vi "Initialize.vi"(7 "Serial Configuration":T1={"Baud Rate"=9600, "Parity"=0, "Data Bits"=8, "Stop Bits"=10, "Flow Control"=0} {"Flow Control" items=["None", "XON/XOFF", "RTS/CTS", "XON/XOFF & RTS/CTS", "DTR/DSR", "XON/XOFF & DTR/DSR"]; "Stop Bits" items=["1.0"=10, "1.5"=15, "2.0"=20]; "Data Bits" items=["7"=7, "8"=8]; "Parity" items=["None", "Odd", "Even", "Mark", "Space"]; "Baud Rate" items=["300"=300, "600"=600, "1200"=1200, "2400"=2400, "4800"=4800, "9600"=9600, "19200"=19200]}, 8 "error in (no error)":errorcluster, 10 "ID Query (True)":bool=TRUE, 11 "VISA resource name":refnum<visa-resource-name>) -> (0 "error out":errorcluster, 3 "VISA resource name out":refnum<visa-resource-name>)   [LabVIEW 2015, in "Samwontech TEMP2xxx.lvlib"]
doc: "Establishes communication with the instrument and optionally performs an instrument identification query and/or an instrument reset. It also places the instrument in a default state needed for other instrument driver operations. Therefore, call this VI before calling other instrument driver VIs for this instrument. Generally, you need to call the <b>Initialize</b> VI only once at the beginning of an application."
uses:
  Samwontech TEMP2xxx.lvlib
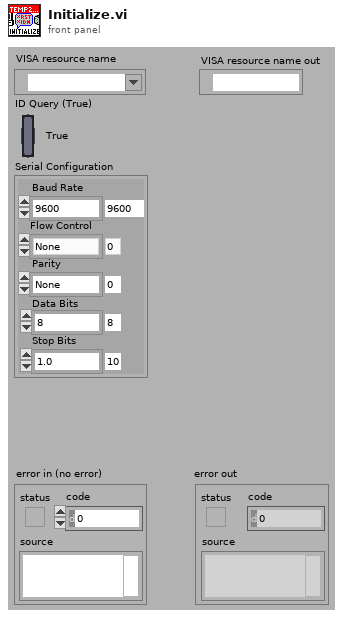
[diagram p1: front panel]
types:
  T1 = cluster{"Baud Rate":u32, "Parity":u16, "Data Bits":u16, "Stop Bits":u16, "Flow Control":u16}
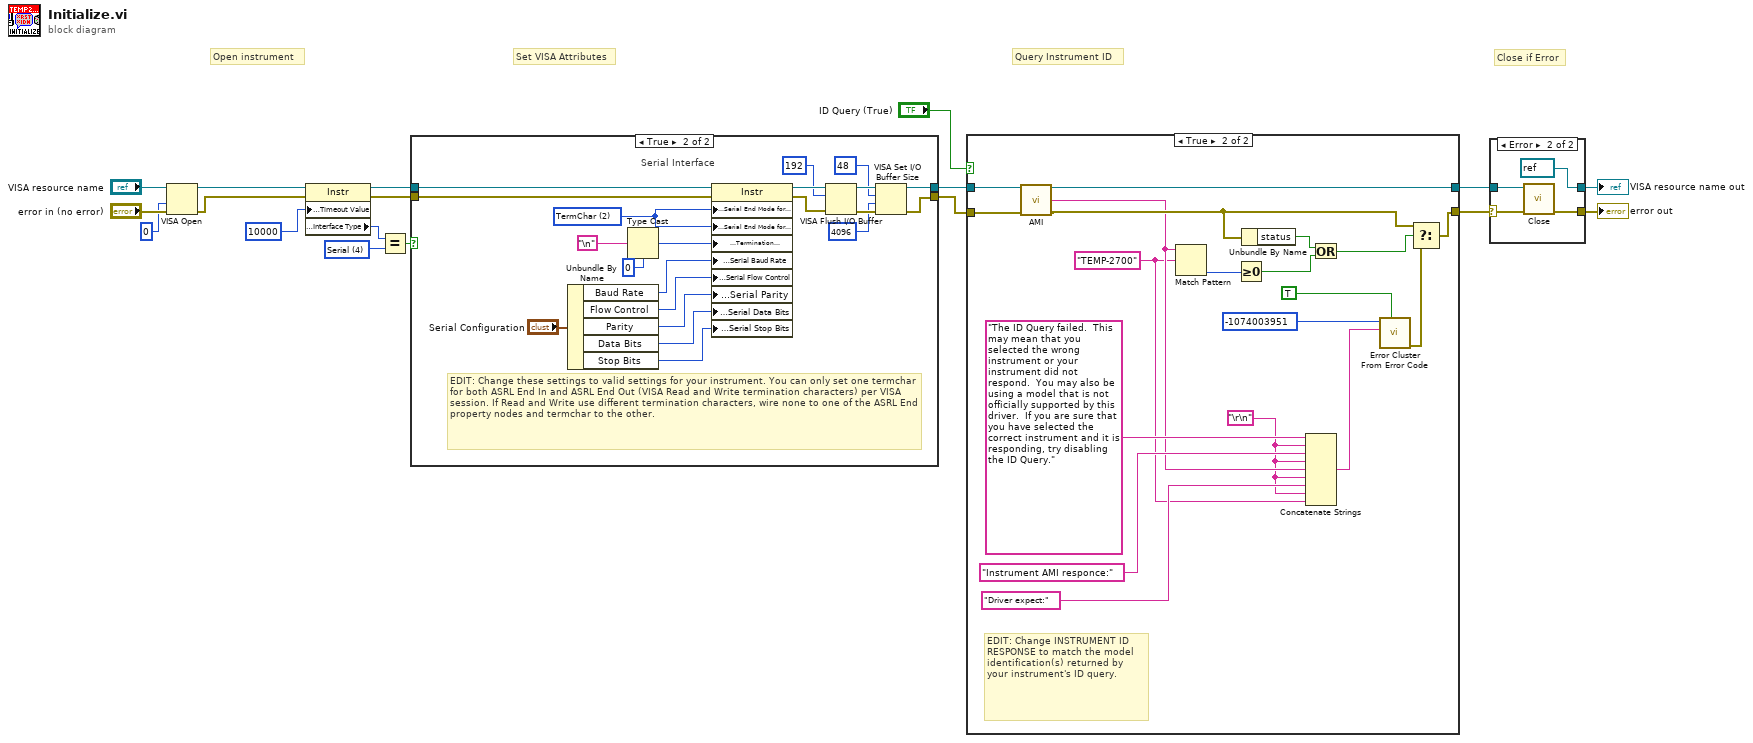
[diagram p0: block diagram]
diagram:
  w6 = u16 4 items=["GPIB"=1, "VXI"=2, "GPIB-VXI"=3, "Serial"=4, "PXI"=5, "TCPIP"=6, "USB"=7] ("Interface Information:Interface Type")
  # "Set VISA Attributes"
  # "Close if Error"
  # "Query Instrument ID"
  # "Open instrument"
  n1 = VISA Open(access mode=u32 0, error in (no error)="error in (no error)", VISA resource name="VISA resource name") -> (VISA resource name=w4:refnum<visa-resource-name>, error out=w3:errorcluster)  [unwired: 2 in]
  n2 = property class="Instr"(reference=w4, error in=w3, "General Settings:Timeout Value"=u32 10000) -> (reference out=w9:refnum<visa-resource-name>, error out=w8:errorcluster, "Interface Information:Interface Type"=w13:u16)
  n3 = Equal?(x=w13, y=w6) -> (x = y?=w7:bool)
  n4 = case shown="True" w7 {
    tunnel: [w19 w38] -> w11
    tunnel: [w20 w35] -> w10
    tunnel: w9 -> [w19 w40]
    tunnel: w8 -> [w20 w41]
    frame False {
      # "EDIT: Remove interfaces not supported by your instrument."
      # "GPIB, TCP/IP, and USB Interface"
    }
    frame True {
      w29 = u16 2 items=["None", "LastBit", "TermChar"] ("Serial Settings:Serial End Mode for Reads")
      # "EDIT: Change these settings to valid settings for your instrument. You can only set one termchar for both ASRL End In and ASRL End Out (VISA Read and Write termination characters) per VISA session. If Read and Write use different termination characters, wire none to one of the ASRL End property nodes and termchar to the other."
      # "Serial Interface"
      n5 = Unbundle By Name("Serial Configuration") -> ("Baud Rate"=w27:u32, "Flow Control"=w23:u16, "Parity"=w25:u16, "Data Bits"=w26:u16, "Stop Bits"=w22:u16)
      n6 = Type Cast(type=u8 0, x="\n") -> (*(type *) &x=w28:u8)
      n7 = property class="Instr"(reference=w40, error in=w41, "Serial Settings:Serial End Mode for Reads"=w29, "Serial Settings:Serial End Mode for Writes"=w29, "Message Based Settings:Termination Character"=w28, "Serial Settings:Serial Baud Rate"=w27, "Serial Settings:Serial Flow Control"=w23, "Serial Settings:Serial Parity"=w25, "Serial Settings:Serial Data Bits"=w26, "Serial Settings:Serial Stop Bits"=w22) -> (reference out=w34:refnum<visa-resource-name>, error out=w37:errorcluster)
      n8 = VISA Flush I/O Buffer(VISA resource name=w34, mask (16)=u16 192, error in (no error)=w37) -> (VISA resource name out=w39:refnum<visa-resource-name>, error out=w36:errorcluster)
      n9 = VISA Set I/O Buffer Size(VISA resource name=w39, mask (16)=u16 48, size (4096)=u32 4096 ("size (0)"), error in (no error)=w36) -> (VISA resource name out=w38:refnum<visa-resource-name>, error out=w35:errorcluster)
    }
  }
  n10 = case shown="True" "ID Query (True)" {
    tunnel: [w42 w62] -> w17
    tunnel: [w43 w52] -> w18
    tunnel: w11 -> [w43 w54]
    tunnel: w10 -> [w42 w53]
    frame False {
    }
    frame True {
      w45 = "\r\n"
      w44 = "TEMP-2700"
      # "EDIT: Change INSTRUMENT ID RESPONSE to match the model identification(s) returned by your instrument's ID query."
      n11 = call "AMI.vi"("VISA resource name"=w54, "error in"=w53) -> ("VISA resource name out"=w52:refnum<visa-resource-name>, "Model Name"=w48:string, "error out"=w51:errorcluster)  [unwired: 8 in, 3 out]
      n12 = Match Pattern(string=w48, regular expression=w44) -> (offset past match=w58:i32)  [unwired: 1 in, 3 out]
      n13 = Greater Or Equal To 0?(x=w58) -> (x >= 0?=w56:bool)
      n14 = Unbundle By Name(w51) -> ("status"=w57:bool)
      n15 = Concatenate Strings("The ID Query failed.  This may mean that you selected the wrong instrument or your instrument did not respond.  You may also be using a model that is not officially supported by this driver.  If you are sure that you have selected the correct instrument and it is responding, try disabling the ID Query." ("Source (VI Name)"), w45, "Instrument AMI responce:", w45, w48, w45, "Driver expect:", w45, w44) -> (w47:string)
      n16 = Or(x=w57, y=w56) -> (x .or. y?=w55:bool)
      n17 = call <vilib>:"Error Cluster From Error Code.vi"("show call chain? (False)"=TRUE, "error message (\"\")"=w47, "error code (0)"=-1074003951 ("Code")) -> ("error out"=w61:errorcluster)  [unwired: 6 in]
      n18 = Select(t=w51, s=w55, f=w61) -> (s? t:f=w62:errorcluster)
    }
  }
  n19 = case shown="Error" w17 {
    selector: w17 -> [w63 w66]
    tunnel: w18 -> [w64 w67]
    tunnel: [w64 refnum<visa-resource-name> refnum ("VISA resource name out")] -> w1
    tunnel: [w63 w68] -> w2
    frame No Error {
    }
    frame Error {
      n20 = call "Close.vi"("error in (no error)"=w66, "VISA resource name"=w67) -> ("error out"=w68:errorcluster)  [unwired: 9 in]
    }
  }
  "error out" <- w2
  "VISA resource name out" <- w1
